vi "URI from Host Port.vi"(7 "Scheme (tcp)":string="tcp", 10 "Port":u16, 11 "Host":string) -> (3 "URI":refnum<class "URI.lvclass">)   [LabVIEW 2020, in "Stream-TCP.lvlib"]
uses:
  Stream-TCP.lvlib
  lv-stream/stream/URI/URI.lvclass
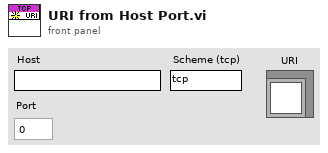
[diagram p1: front panel]
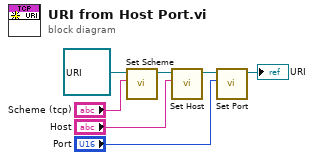
[diagram p0: block diagram]
diagram:
  n1 = call "Set Scheme.vi"("Scheme"="Scheme (tcp)", "URI in"=refnum<class "URI.lvclass"> refnum ("Stream.lvlib:URI.lvclass")) -> ("URI out"=w6:refnum<class "URI.lvclass">)  [unwired: 8 in, 1 out]
  n2 = call "Set Host.vi"("Host"="Host", "URI in"=w6) -> ("URI out"=w5:refnum<class "URI.lvclass">)  [unwired: 8 in, 1 out]
  n3 = call "Set Port.vi"("Port"="Port", "URI in"=w5) -> ("URI out"=→"URI":refnum<class "URI.lvclass">)  [unwired: 8 in, 1 out]
